vi "Get Mecanum Wheel Click Zones.vi"(7 "global wheel position":cluster{"x":dbl, "y":dbl}, 8 "error in (no error)":errorcluster, 9 "wheel index":i32, 11 "wheel in":refnum<class "NI_Robotics_Wheel.lvclass">) -> (0 "error out":errorcluster, 2 "click zones":T1[](array[typedef]), 3 "wheel out":refnum<class "NI_Robotics_Wheel.lvclass">)   [LabVIEW 2017, in "NI_Robotics_Configure Steering Frame.lvlib"]
uses:
  <vilib>/robotics/Dialog/Configure Steering Frame/NI_Robotics_Configure Steering Frame.lvlib
  <vilib>/robotics/Dialog/Configure Steering Frame/Click Zone.ctl
  <vilib>/robotics/Steering/Wheel/NI_Robotics_Wheel.lvclass
  <vilib>/robotics/Steering/Wheel/Get Mecanum Wheel Information.vi
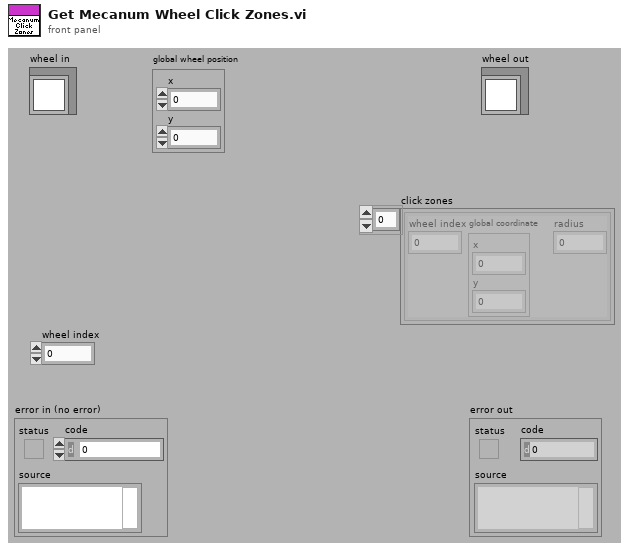
[diagram p1: front panel]
types:
  T1 = typedef "NI_Robotics_Configure Steering Frame.lvlib/Click Zone.ctl" = cluster{"wheel index":i32, "global coordinate":cluster{"x":dbl, "y":dbl}, "radius":dbl}
  T2 = typedef "NI_Robotics_Wheel.lvclass/Wheel Parameters.ctl" = cluster{"wheel radius":dbl, "gear ratio":dbl, "forward rotation direction":T3}
  T3 = typedef "NI_Robotics_Wheel.lvclass/Rotation Direction.ctl" = u16
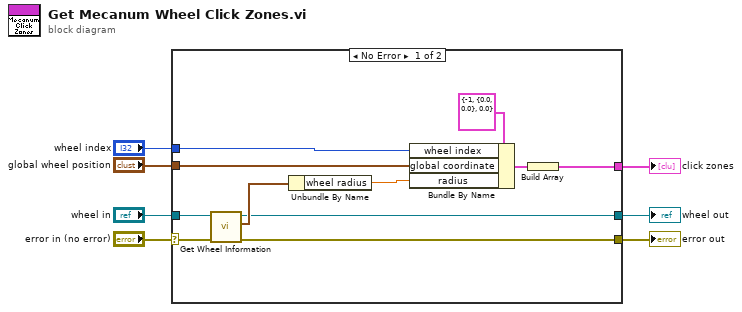
[diagram p0: block diagram]
diagram:
  n1 = case shown="No Error" "error in (no error)" {
    selector: "error in (no error)" -> [w17 w20]
    tunnel: [w16 w20] -> w5
    tunnel: "wheel in" -> [w18 w19]
    tunnel: "global wheel position" -> [w10 _]
    tunnel: [w14 w19] -> w4
    tunnel: "wheel index" -> [w12 _]
    tunnel: [w11 _] -> w7
    frame No Error {
      n2 = call-poly <vilib>:"Get Wheel Information.vi"("error in (no error)"=w17, "wheel in"=w18) -> ("error out"=w16:errorcluster, "wheel parameters"=w15:T2, "wheel out"=w14:refnum<class "NI_Robotics_Wheel.lvclass">)  [unwired: 4 in, 3 out]
      n3 = Unbundle By Name(w15) -> ("wheel radius"=w9:dbl)
      n4 = Bundle By Name(cluster=T1 {"wheel index"=-1, "global coordinate"={"x"=0.0, "y"=0.0}, "radius"=0.0} ("click zone"), "wheel index"=w12, "global coordinate"=w10, "radius"=w9) -> (w13:T1)
      n5 = Build Array(w13) -> (w11:T1[])
    }
    frame Error {
    }
  }
  "error out" <- w5
  "wheel out" <- w4
  "click zones" <- w7
